vi "Sort Mapping parameters metadata.vi"(0 "reference in":refnum<class "metadata.lvclass">, 5 "error in (no error)":errorcluster) -> (14 "reference out":refnum<class "metadata.lvclass">, 16 "Mapping":T1, 19 "error out":errorcluster)   [LabVIEW 2019, in "metadata.lvclass"]
uses:
  metadata.lvclass
  Mapping parameters.ctl
panel:
  out "Array":string[](array[string])
  out "Array 2":i32[](array[numeric])
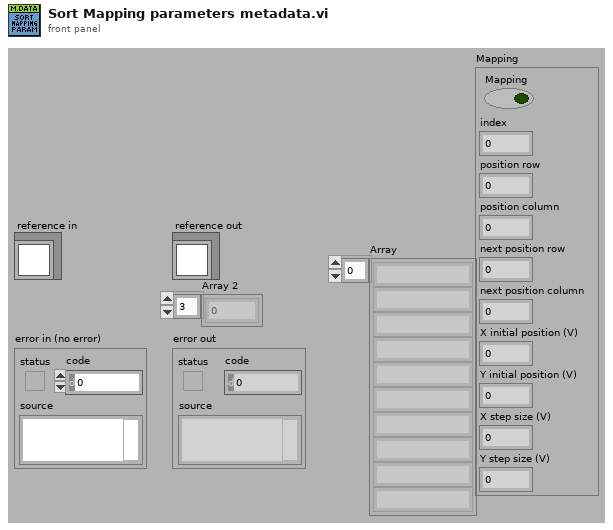
[diagram p1: front panel]
types:
  T1 = typedef "metadata.lvclass/Mapping parameters.ctl" = cluster{"Mapping":bool, "index":u16, "position row":u16, "position column":u16, "next position row":i16, "next position column":i16, "X initial position (V)":dbl, "Y initial position (V)":dbl, "X step size (V)":dbl, "Y step size (V)":dbl}
  T2 = typedef "metadata.lvclass/ObjectAttributesRef.ctl" = refnum<data-value>
  T3 = typedef "metadata.lvclass/ObjectAttributes.ctl" = cluster{"MyAttribute":dbl, "System Control":T4, "file info":T5, "Sample info":T6, "Cantilever info":T7, "XYZ piezos":T8, "Mapping":T1, "Fcurve segment":T9[], "Fast fpga segment":T11, "Chirp":T12, "precision (6)":i16, "width (-)":i16, "Metadata":T13, "config filepath":path, "Section names []":string[], "Property names []":string[], "nb elements":u16}
  T4 = typedef "metadata.lvclass/System control parameters.ctl" = cluster{"FPGA SW version":string, "TDMS file version":string, "Instrument":string, "Instrument model":string, "Instrument scanner":string, "Instrument clockrate (Mhz)":string, "Instrument tick time (us)":string}
  T5 = typedef "metadata.lvclass/File info parameters.ctl" = cluster{"Time Stamp":timestamp, "Filename":string, "Filepath":path, "User":string, "Experiment_name":string, "Curve_id":string, "number_segments":u8, "number_consecutive_scans":u32}
  T6 = typedef "metadata.lvclass/Sample info parameters.ctl" = cluster{"Sample name":string, "Sample species":string}
  T7 = typedef "metadata.lvclass/Cantilever info parameters.ctl" = cluster{"spring constant calib method":string, "invOLS calib method":string, "thermal calib deflection channel":string, "model":string, "shape":string, "tip geometry":string, "Laser sum (V)":dbl, "Laser power (mA)":dbl, "invOLS_(nm/V)":dbl, "spring constant nominal (N/m)":dbl, "spring constant calib (N/m)":dbl, "resosnance frequency air calib (Hz)":dbl, "resosnance frequency calib (Hz)":dbl, "quality factor":dbl, "Acoefficident_GCI_(nN.s^1.3/m)":dbl, "half angle (deg)":dbl, "tip radius (m)":dbl, "tip height (m)":dbl, "system mount angle (deg)":dbl}
  T8 = typedef "metadata.lvclass/XYZ piezos parameters.ctl" = cluster{"X stage piezo sensitivity (nm/V)":dbl, "X stage piezo gain":dbl, "X velocity (V/tick)":dbl, "X closed loop":bool, "Y stage piezo sensitivity (nm/V)":dbl, "Y stage piezo gain":dbl, "Y velocity (V/tick)":dbl, "Y closed loop":bool, "Z stage piezo sensitivity (nm/V)":dbl, "Z stage piezo gain":dbl, "Z closed loop":bool, "X position (V)":dbl, "Y position (V)":dbl}
  T9 = typedef "metadata.lvclass/Fcurve segment.ctl" = cluster{"type":T10, "fast_fpga_trigger":bool, "nb":u8, "duration (ticks)":i64, "nb points":i32, "sampling rate (S/s)":u32, "Zpiezo control out":string, "initial deflection (V)":dbl, "relative setpoint":bool, "setpoint on":bool, "setpoint (V)":dbl, "setpoint trigger channel":string, "velocity (V/tick)":dbl, "Z position setpoint trigger (V)":dbl, "Z retract length (V)":dbl, "dec factor":u32}
  T10 = typedef "metadata.lvclass/Segment type--combobox.ctl" = string
  T11 = typedef "metadata.lvclass/fast fpga segment parameters.ctl" = cluster{"Fast start time trigger":timestamp, "nb_points":u32, "sampling_rate_(S/s)":u32, "duration_(ticks)":u32}
  T12 = typedef "metadata.lvclass/Chirp added parameters.ctl" = cluster{"f start (Hz)":dbl, "f end (Hz)":dbl, "Sweep type":string}
  T13 = typedef "metadata.lvclass/Metadata output --cluster.ctl" = cluster{"Property Names":string[], "Property Values":variant[]}
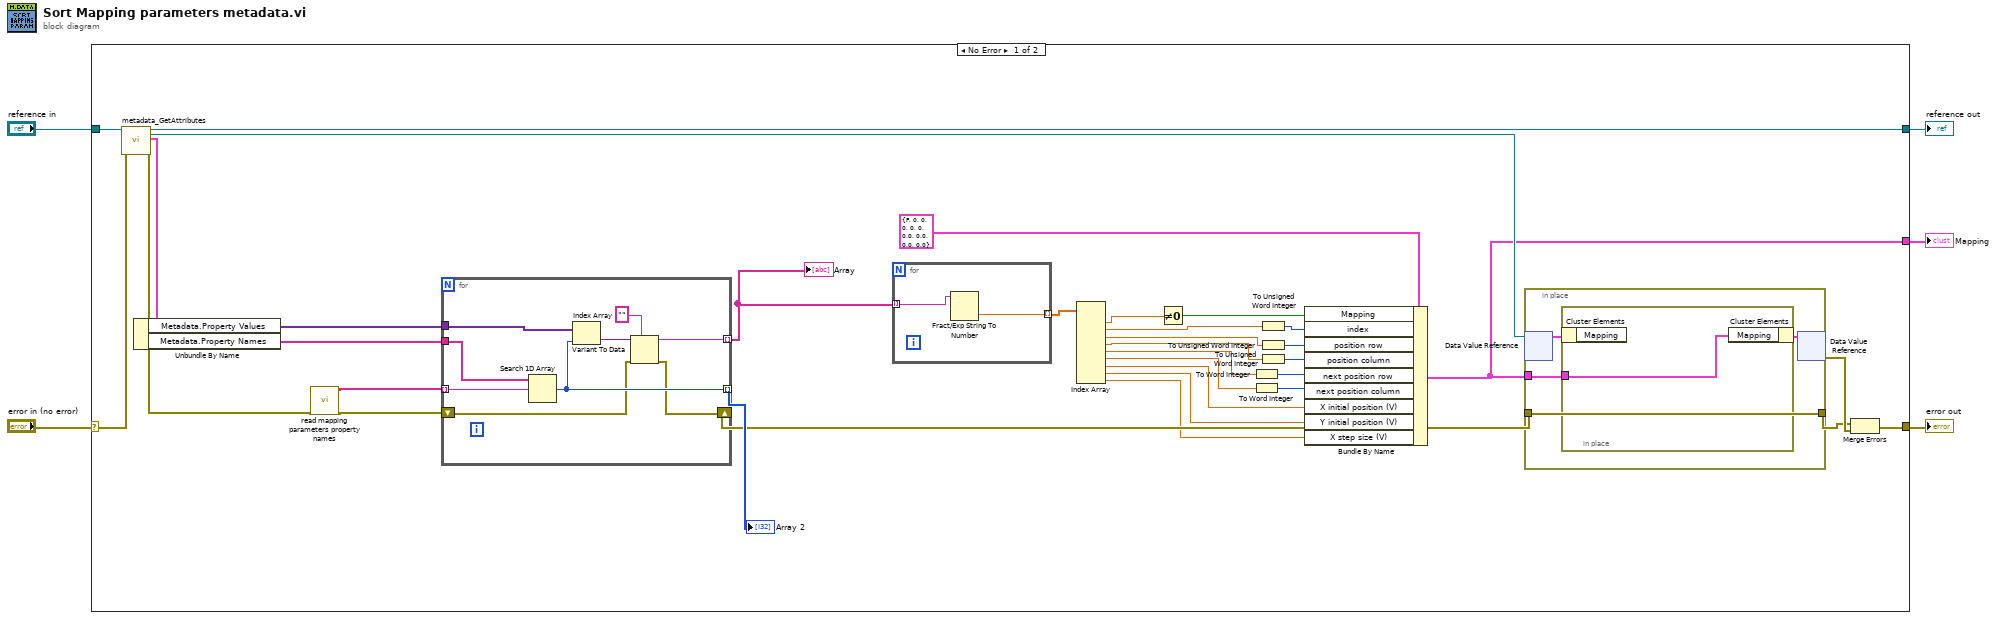
[diagram p0: block diagram]
diagram:
  n1 = case shown="No Error" "error in (no error)" {
    selector: "error in (no error)" -> [w35 w57]
    tunnel: [w39 w57] -> w4
    tunnel: [w34 w56] -> w2
    tunnel: "reference in" -> [w36 w56]
    tunnel: [w27 _] -> w1
    frame No Error {
      n2 = call "metadata_GetAttributes.vi"("reference in"=w36, "error in (no error)"=w35) -> ("reference out"=w34:refnum<class "metadata.lvclass">, "attributes ref"=w33:T2, "attributes"=w32:T3, "error out"=w24:errorcluster)  [unwired: 14 in]
      n3 = Unbundle By Name(w32) -> ("Metadata.Property Values"=w28:variant[], "Metadata.Property Names"=w31:string[])
      n4 = call "read mapping parameters property names.vi"("error in (no error)"=w24) -> ("Mapping param"=w22:string[], "error out"=w23:errorcluster)  [unwired: 17 in]
      n5 = for {
        tunnel: w22 -> [w50] mode=indexing
        tunnel: [w47] -> w30 mode=indexing
        shift-right: [w43] -> w29
        shift-left: w23 -> [w44]
        tunnel: w31 -> [w49]
        tunnel: w28 -> [w48]
        tunnel: [w45] -> w25 mode=indexing
        n6 = Search 1D Array(1D array=w49, element=w50) -> (index of element=w47:i32)  [unwired: 1 in]
        n7 = Index Array(array=w48, index=w47) -> (element=w46:variant)
        n8 = Variant To Data(error in=w44, type="", Variant=w46) -> (data=w45:string, error out=w43:errorcluster)
      }
      "Array 2" <- w30
      "Array" <- w25
      n9 = for {
        tunnel: [w41] -> w26 mode=indexing
        tunnel: w25 -> [w40] mode=indexing
        n10 = Fract/Exp String To Number(string=w40) -> (number=w41:dbl)  [unwired: 3 in, 1 out]
      }
      n11 = Index Array(array=w26) -> (element #1=w20:dbl, element #2=w18:dbl, element #3=w12:dbl, element #4=w11:dbl, element #5=w10:dbl, element #6=w9:dbl, element #7=w8:dbl, element #8=w7:dbl, element #9=w6:dbl)  [unwired: 9 in]
      n12 = Not Equal To 0?(x=w20) -> (x != 0?=w19:bool)
      n13 = To Word Integer(number=w10) -> (16bit integer=w14:i16)
      n14 = To Word Integer(number=w9) -> (16bit integer=w13:i16)
      n15 = To Unsigned Word Integer(number=w18) -> (unsigned 16bit integer=w17:u16)
      n16 = To Unsigned Word Integer(number=w12) -> (unsigned 16bit integer=w16:u16)
      n17 = To Unsigned Word Integer(number=w11) -> (unsigned 16bit integer=w15:u16)
      n18 = Bundle By Name(cluster=T1 {"Mapping"=FALSE, "index"=0, "position row"=0, "position column"=0, "next position row"=0, "next position column"=0, "X initial position (V)"=0.0, "Y initial position (V)"=0.0, "X step size (V)"=0.0, "Y step size (V)"=0.0} ("Mapping"), "Mapping"=w19, "index"=w17, "position row"=w16, "position column"=w15, "next position row"=w14, "next position column"=w13, "X initial position (V)"=w8, "Y initial position (V)"=w7, "X step size (V)"=w6) -> (w27:T1)
      n19 = in-place {
        in-place-border: w29 -> [w52]
        in-place-border: [w52] -> w37
        in-place-border: w27 -> [w51]
        n20 = in-place-dvr #1(w33) -> (w53:T3)  [unwired: 1 out]
        n21 = in-place {
          in-place-border: w51 -> [w55]
          n22 = in-place-cluster #2(w53) -> ()  [unwired: 1 out]
          n23 = in-place-cluster #2("Mapping"=w55) -> (w54:T3)
        }
        n24 = in-place-dvr #1(w54) -> (w38:errorcluster)  [unwired: 1 out]
      }
      n25 = Merge Errors(w37, w38) -> (w39:errorcluster)
    }
    frame Error {
    }
  }
  "error out" <- w4
  "reference out" <- w2
  "Mapping" <- w1
